vi "ESA-C Position to Voltage v10.5.2.vi"(1 "Axis":i32, 2 "Position (µm)":dbl) -> (0 "Voltage (V)":dbl)   [LabVIEW 2010]
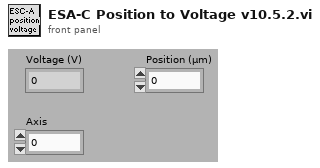
[diagram p1: front panel]
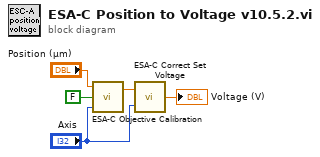
[diagram p0: block diagram]
diagram:
  n1 = call "ESA-C Objective Calibration.vi"("Axis"="Axis", "Is Voltage?"=FALSE, "Input Value"="Position (µm)") -> ("Output Value"=w3:dbl)  [unwired: 1 in]
  n2 = call "ESA-C Correct Set Voltage.vi"("Axis"="Axis", "Target Voltage (V)"=w3) -> ("Command Voltage (V)"=→"Voltage (V)":dbl)
